vi "Set Server Certificate File.vi"(10 "Server Certificate File (.crt)":path, 11 "OOP Server in":refnum<class "Temperature_server.lvclass">) -> (3 "OOP Server out":refnum<class "Temperature_server.lvclass">)   [LabVIEW 2019, in "Temperature_server.lvlib" / "Temperature_server.lvclass"]
uses:
  Temperature_server.lvclass
  Temperature_server.lvclass/Temperature_server.ctl
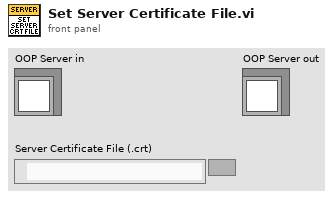
[diagram p1: front panel]
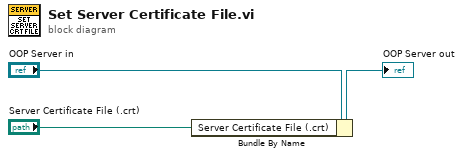
[diagram p0: block diagram]
diagram:
  n1 = Bundle By Name(cluster="OOP Server in", "Server Certificate File (.crt)"="Server Certificate File (.crt)") -> (→"OOP Server out":refnum<class "Temperature_server.lvclass">)
